vi "update channel config path in user config.vi"(9 "messageHandler in":T1 {"params"."controlChannels"."ballControl" items=["Module6/output0", "Module6/output1", "Module6/output2", "Module6/output3", "Not-Used"]; "params"."controlChannels"."butterflyControl" items=["Module6/output0", "Module6/output1", "Module6/output2", "Module6/output3", "Not-Used"]; "params"."controlChannels"."speedControl" items=["Module6/output0", "Module6/output1", "Module6/output2", "Module6/output3", "Not-Used"]}, 10 "new path":variant, 11 "Queues in":T2) -> ()   [LabVIEW 2018]
uses:
  type defs/Queues.ctl
  type defs/message handler data.ctl
  customVI/liveData/state.ctl
  supporting VIs/polymorphic VIs/enqueue for user interface.vi
  <vilib>/Utility/config.llb/Write Key (Path).vi
  <vilib>/Utility/config.llb/NI_LVConfig.lvlib
panel:
  out "new channel config path":path
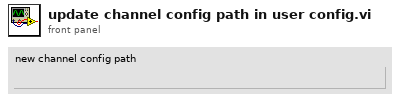
[diagram p1: front panel]
types:
  T1 = typedef "message handler data.ctl" = cluster{"params":cluster{"configFileID":u32, "configFilePath":path, "channelConfigFilePath":path, "incidentLogfile":path, "controlChannels":cluster{"ballControl":u16, "butterflyControl":u16, "speedControl":u16}, "pulsatorVIPath":path, "customVIPath":path, "HowdenAir":cluster{"vent Howden":bool, "Howden%":dbl}}, "vars":cluster{"commsStatus":bool[], "controlIndex":cluster{"ballControl":u16, "butterflyControl":u16, "speedControl":u16}, "customVIRef":refnum<vi>, "Interlocks":cluster{"gearboxOil":bool, "bearingOil":bool, "gearboxAir":bool}, "motorRunning":bool, "liveDataQ":refnum<queue>[]}}
  T2 = typedef "Queues.ctl" = cluster{"messageHandler":refnum<queue>, "comms":refnum<queue>, "dataStream":refnum<queue>, "dataProcessor":refnum<queue>, "fileIO":refnum<queue>, "userInterface":refnum<queue>, "errors":refnum<queue>, "customCompressor":refnum<queue>}
  T3 = typedef "NI_LVConfig.lvlib/Config Data RefNum.ctl" = refnum<k1>
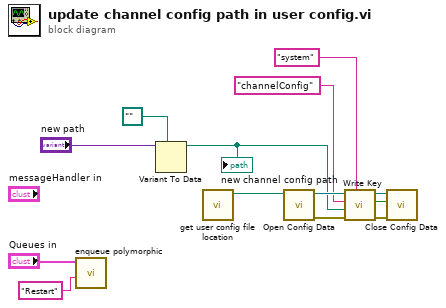
[diagram p0: block diagram]
diagram:
  n1 = call-poly "enqueue polymorphic.vi"("message"="Restart", "Queues"="Queues in") -> ()  [unwired: 9 in, 1 out]
  n2 = Variant To Data(type=path "", Variant="new path") -> (data=w4:path)  [unwired: 1 in, 1 out]
  "new channel config path" <- w4
  n3 = call "get user config file location.vi"() -> ("userConfigPath"=w1:path)  [unwired: 11 in]
  n4 = call <vilib>:"Open Config Data.vi"("configuration file path"=w1) -> ("error out"=w11:errorcluster, "refnum"=w10:T3)  [unwired: 8 in, 1 out]
  n5 = call-poly <vilib>:"Write Key.vi"("section"="system", "error in (no error)"=w11, "value"=w4, "key"="channelConfig", "refnum"=w10) -> ("error out"=w7:errorcluster, "found?"=w6:bool, "refnum out"=w5:T3)  [unwired: 4 in]
  n6 = call <vilib>:"Close Config Data.vi"("error in (no error)"=w7, "write file if changed (T)"=w6, "refnum"=w5) -> ()  [unwired: 7 in, 2 out]
